vi "test Get TagDistance By TagID.vi"(8 "error in (no error)":errorcluster, 11 "TestCase in":refnum<class "AnchorTests.lvclass">) -> (0 "error out":errorcluster, 3 "TestCase out":refnum<class "AnchorTests.lvclass">)   [LabVIEW 2014, in "AnchorTests.lvclass"]
uses:
  AnchorTests.lvclass
  <vilib>/addons/_JKI Toolkits/VI Tester/TestCase.llb/TestCase.lvclass
  SPLAT/Tag.lvclass
  SPLAT/Anchor/Anchor.lvclass
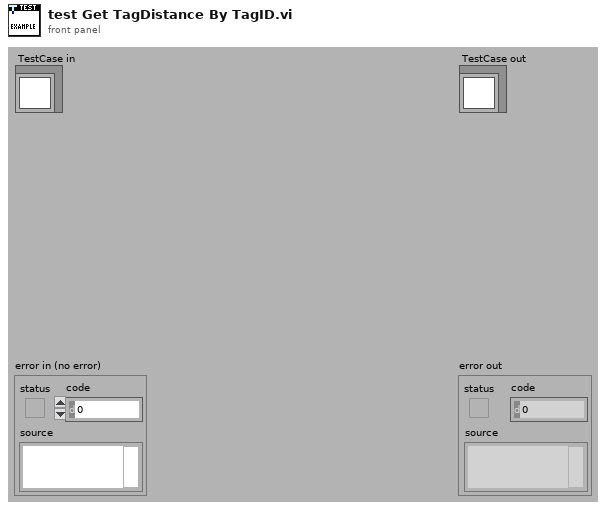
[diagram p1: front panel]
types:
  T1 = cluster{"Tag Out":refnum<class "Tag.lvclass">, "TagY":dbl}
  T2 = cluster{"Tag Out":refnum<class "Tag.lvclass">, "TagY":dbl}[]
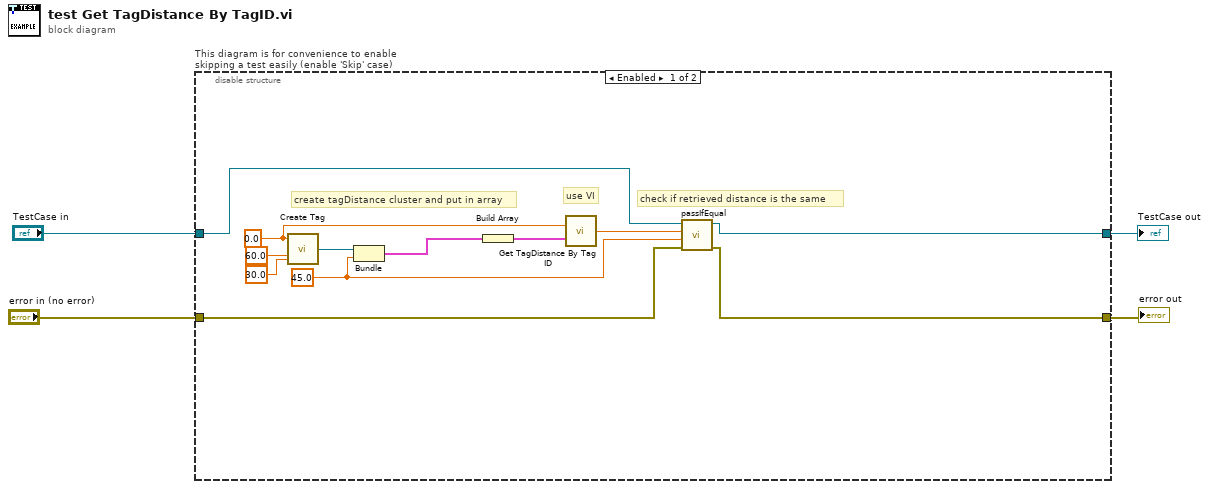
[diagram p0: block diagram]
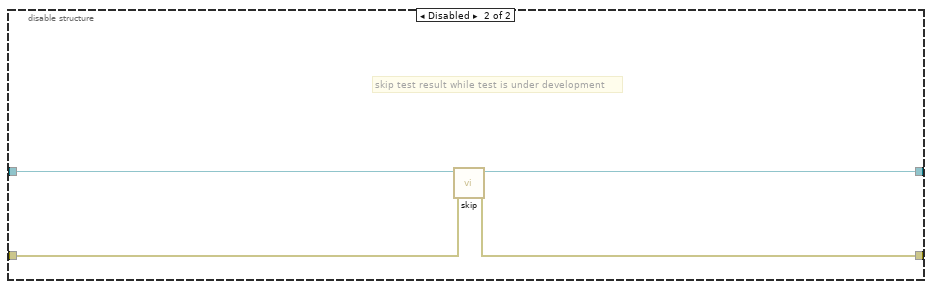
[diagram p2: hidden frame]
diagram:
  n1 = disable-structure "This diagram is for convenience to enable skipping a test easily (enable 'Skip' case)" shown="Enabled" {
    disable-tunnel: "TestCase in" -> [w7 w20]
    disable-tunnel: [w6 w18] -> w1
    disable-tunnel: [w5 w19] -> w3
    disable-tunnel: "error in (no error)" -> [w8 w17]
    frame Enabled {
      w9 = 45.0 ("TagY")
      w11 = 0.0 ("TagID")
      # "check if retrieved distance is the same"
      # "use VI"
      # "create tagDistance cluster and put in array"
      n2 = call "Create Tag.vi"("TagY"=30.0, "TagX"=60.0, "TagID"=w11) -> ("Tag Out"=w14:refnum<class "Tag.lvclass">)
      n3 = Bundle("Tag Out"=w14, "TagY"=w9) -> (w13:T1)  [unwired: 1 in]
      n4 = Build Array(w13) -> (w12:T2)
      n5 = call "Get TagDistance By Tag ID.vi"("TagID"=w11, "TagDistanceArray"=w12) -> ("Distance"=w10:dbl)  [unwired: 13 in]
      n6 = call-dynamic "passIfEqual.vi"("error in (no error)"=w8, "y"=w9, "x"=w10, "TestCase in"=w7) -> ("error out"=w5:errorcluster, "TestCase out"=w6:refnum<class "AnchorTests.lvclass">)  [unwired: 6 in]
    }
    frame Disabled {
      # "skip test result while test is under development"
      n7 = call <vilib>:"skip.vi"("error in (no error)"=w17, "TestCase in"=w20) -> ("error out"=w19:errorcluster, "TestCase out"=w18:refnum<class "AnchorTests.lvclass">)  [unwired: 8 in]
    }
  }
  "error out" <- w3
  "TestCase out" <- w1
